vi "getInfo_action.vi"(0 "HGF_ImaqFg":refnum<class "HGF_ImaqFg.lvclass">, 5 "error in (no error)":errorcluster) -> (13 "imageType":T1 items=["Grayscale (U8)", "Grayscale (I16)", "Grayscale (SGL)", "Complex (CSG)", "RGB (U32)", "HSL (U32)", "RGB (U64)", "Grayscale (U16)"], 14 "dup HGF_ImaqFg":refnum<class "HGF_ImaqFg.lvclass">, 15 "cameraName":string, 16 "controlMode":T2, 17 "videoMode":i32, 19 "error out":errorcluster)   [LabVIEW 2014, in "HGF_IMAQ.lvlib" / "HGF_ImaqFg.lvclass"]
doc: "Return the name of camera."
uses:
  HGF_ImaqFg.lvclass
  HGF_IMAQDevice/HGF_IMAQDevice.lvclass
  HGF_IMAQDevice/Control Mode.ctl
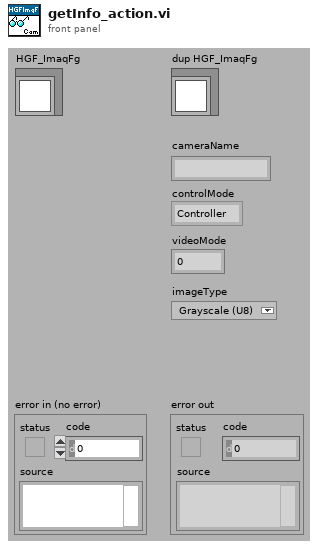
[diagram p1: front panel]
types:
  T1 = typedef "Image Type" = u32
  T2 = typedef "HGF_IMAQ.lvlib/HGF_IMAQDevice.lvclass/Control Mode.ctl" = enum16{"Controller", "Listener"}
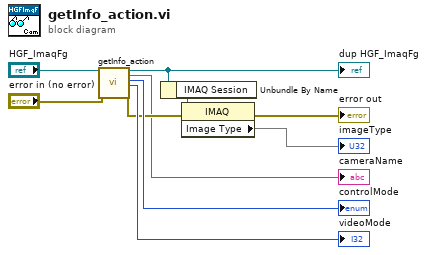
[diagram p0: block diagram]
diagram:
  n1 = call-parent "getInfo_action.vi"("HGF_IMAQDevice"="HGF_ImaqFg", "error in (no error)"="error in (no error)") -> ("dup HGF_IMAQDevice"=w6:refnum<class "HGF_ImaqFg.lvclass">, "cameraName"=→"cameraName":string, "controlMode"=→"controlMode":T2, "videoMode"=→"videoMode":i32, "error out"=w3:errorcluster)  [unwired: 13 out]
  "dup HGF_ImaqFg" <- w6
  n2 = Unbundle By Name(w6) -> ("IMAQ Session"=w5:refnum<k11>)
  n3 = property class="IMAQ"(reference=w5, error in=w3) -> (error out=→"error out":errorcluster, "Image Type"=→"imageType")  [unwired: 1 out]
